vi "Test_AllOnes_AvgEqualsOne.vi"(8 "error in (no error)":errorcluster, 11 "TestCase in":refnum<class "TestTimedAverageBuffer.lvclass">) -> (0 "error out":errorcluster, 3 "TestCase out":refnum<class "TestTimedAverageBuffer.lvclass">)   [LabVIEW 2015, in "TimedAverageBuffer.lvlib" / "TestTimedAverageBuffer.lvclass"]
uses:
  TestTimedAverageBuffer.lvclass
  <vilib>/addons/_JKI Toolkits/VI Tester/TestCase.llb/TestCase.lvclass
  TimedAverageBuffer.lvclass
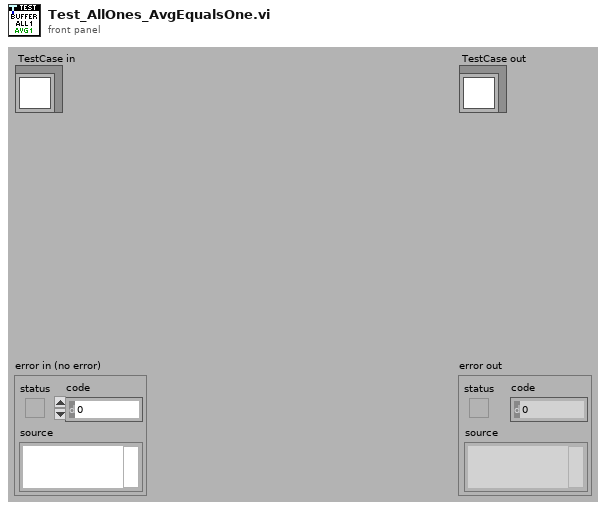
[diagram p1: front panel]
types:
  T1 = typedef "TimedAverageBuffer.lvlib/TimedAverageBuffer.lvclass/TimedAverageBuffer Reference.ctl" = refnum<data-value>
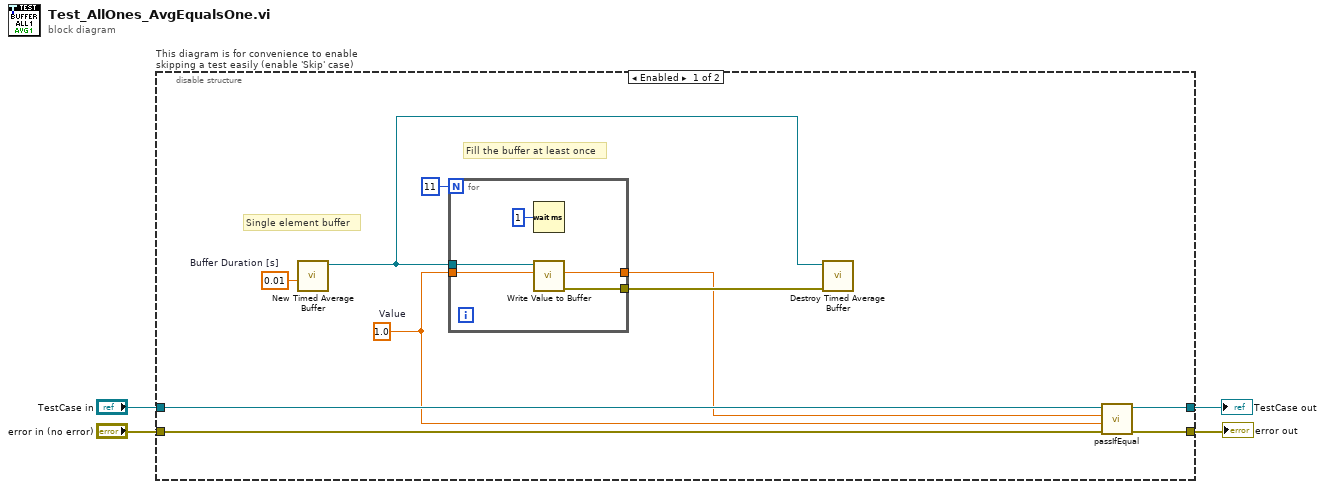
[diagram p0: block diagram]
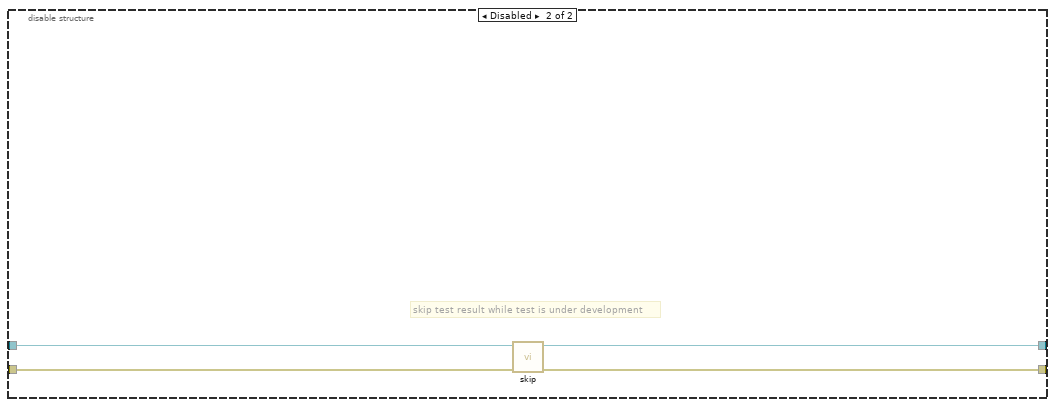
[diagram p2: hidden frame]
diagram:
  n1 = disable-structure "This diagram is for convenience to enable skipping a test easily (enable 'Skip' case)" shown="Enabled" {
    disable-tunnel: "TestCase in" -> [w14 w23]
    disable-tunnel: [w13 w21] -> w1
    disable-tunnel: [w12 w22] -> w3
    disable-tunnel: "error in (no error)" -> [w11 w20]
    frame Enabled {
      w10 = 0.01  # Buffer Duration [s]
      w6 = 1.0  # Value
      # "Fill the buffer at least once"
      # "Single element buffer"
      n2 = call "New Timed Average Buffer.vi"("Buffer Duration [s]"=w10) -> ("Timed Average Buffer"=w9:T1)  [unwired: 9 in, 1 out]
      n3 = for {
        N: 11 -> [_]
        tunnel: w9 -> [w19]
        tunnel: [w18] -> w8
        tunnel: [w15] -> w7
        tunnel: w6 -> [w17]
        n4 = Wait (ms)(milliseconds to wait=u32 1) -> ()  [unwired: 1 out]
        n5 = call "Write Value to Buffer.vi"("Value"=w17, "Timed Average Buffer"=w19) -> ("error out"=w18:errorcluster, "Average"=w15:dbl)  [unwired: 6 in, 2 out]
      }
      n6 = call "Destroy Timed Average Buffer.vi"("error in (no error)"=w8, "Timed Average Buffer"=w9) -> ()  [unwired: 9 in, 1 out]
      n7 = call-dynamic "passIfEqual.vi"("error in (no error)"=w11, "y"=w6, "x"=w7, "TestCase in"=w14) -> ("error out"=w12:errorcluster, "TestCase out"=w13:refnum<class "TestTimedAverageBuffer.lvclass">)  [unwired: 6 in]
    }
    frame Disabled {
      # "skip test result while test is under development"
      n8 = call <vilib>:"skip.vi"("error in (no error)"=w20, "TestCase in"=w23) -> ("error out"=w22:errorcluster, "TestCase out"=w21:refnum<class "TestTimedAverageBuffer.lvclass">)  [unwired: 8 in]
    }
  }
  "error out" <- w3
  "TestCase out" <- w1
